vi "Preprocess_and_Convert_IMAQ_Image_to_Array.vi"(7 "PreProcessing_Options":T2={"DS_Name"="delete", "Input_Dims"={"C"=3, "H"=224, "W"=224}, "Center Crop Size"=0, "Interpolation Type"=1, "Multi-Stage_DownSample?"=FALSE, "Dataset_Stats"={"means"={"R"=0.5385, "G"=0.5348, "B"=0.551}, "stds"={"R"=0.3673, "G"=0.3673, "B"=0.3505}}} {"Dataset_Stats"."stds"."R" format="%#_3g"; "Dataset_Stats"."stds"."G" format="%#_3g"; "Dataset_Stats"."stds"."B" format="%#_3g"; "Dataset_Stats"."means"."R" format="%#_3g"; "Dataset_Stats"."means"."G" format="%#_3g"; "Dataset_Stats"."means"."B" format="%#_3g"; "Interpolation Type" items=["Zero Order", "Bi-Linear", "Quadratic", "Cubic Spline"]}, 8 "error in (no error)":errorcluster, 11 "Imaq Image In":T1=refnum) -> (0 "error out":errorcluster, 2 "Norm_Img_Out":sgl[][][](array[numeric]), 3 "Imaq Image Out":T1, 5 "dT_Preprocessing":dbl=0.0017125000013038516)   [LabVIEW 2024]
uses:
  <vilib>/Ngene/DeepLTK Anomaly Detection Addon/DeepLTK_Anomaly_Detection_Addon/API/Controls/NNPC_PreProcessing_Options.ctl
  <vilib>/Ngene/Deep Learning Toolkit/Toolkit/NN_Data/API/NN_Dims(C,H,W).ctl
  <vilib>/Ngene/DeepLTK Anomaly Detection Addon/DeepLTK_Anomaly_Detection_Addon/API/Controls/NNPC_DS_Stats.ctl
  <vilib>/Ngene/DeepLTK Anomaly Detection Addon/DeepLTK_Anomaly_Detection_Addon/API/Controls/Image_Stats_RGB.ctl
  <vilib>/vision/Image Controls.llb/IMAQ Image.ctl
  <vilib>/vision/NI_Vision_Development_Module.lvlib
  <vilib>/Ngene/Deep Learning Toolkit/Toolkit/Deep_Learning_Toolkit_by_Ngene.lvlib
  <vilib>/Ngene/DeepLTK Anomaly Detection Addon/DeepLTK_Anomaly_Detection_Addon/DeepLTK_Anomaly_Detection_Addon.lvlib
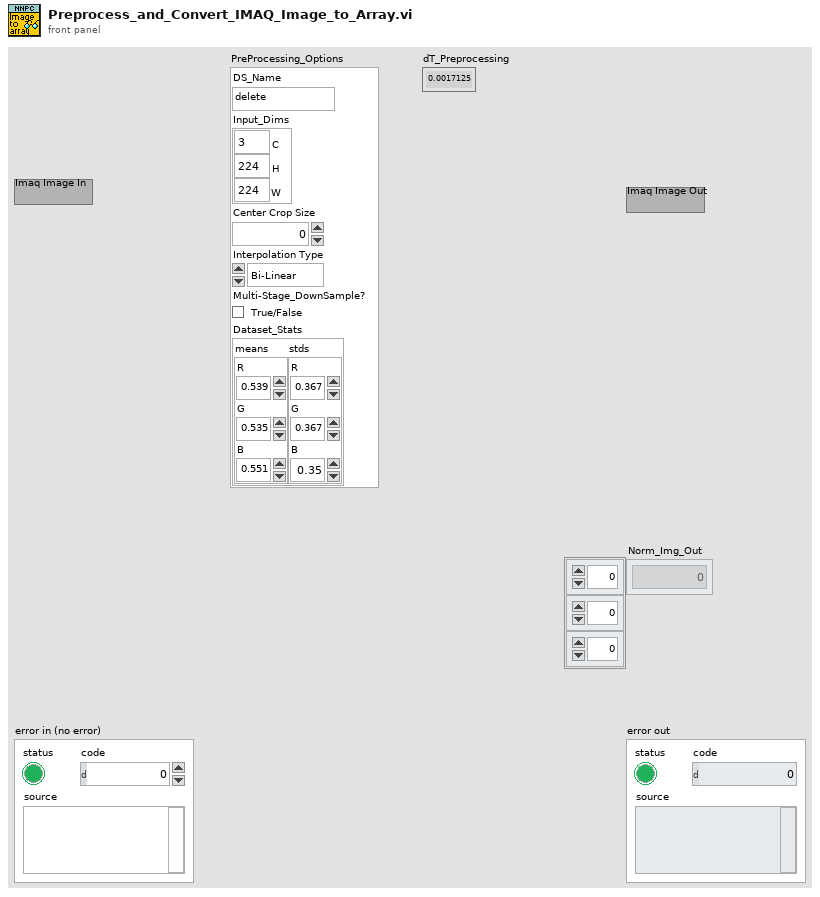
[diagram p1: front panel]
types:
  T1 = typedef "IMAQ Image.ctl" = refnum<image>
  T2 = typedef "DeepLTK_Anomaly_Detection_Addon.lvlib/NNPC_PreProcessing_Options.ctl" = cluster{"DS_Name":string, "Input_Dims":T3, "Center Crop Size":i32, "Interpolation Type":u32, "Multi-Stage_DownSample?":bool, "Dataset_Stats":T4}
  T3 = typedef "Deep_Learning_Toolkit_by_Ngene.lvlib/NN_Dims(C,H,W).ctl" = cluster{"C":i32, "H":i32, "W":i32}
  T4 = typedef "DeepLTK_Anomaly_Detection_Addon.lvlib/NNPC_DS_Stats.ctl" = cluster{"means":T5, "stds":T5}
  T5 = typedef "DeepLTK_Anomaly_Detection_Addon.lvlib/Image_Stats_RGB.ctl" = cluster{"R":sgl, "G":sgl, "B":sgl}
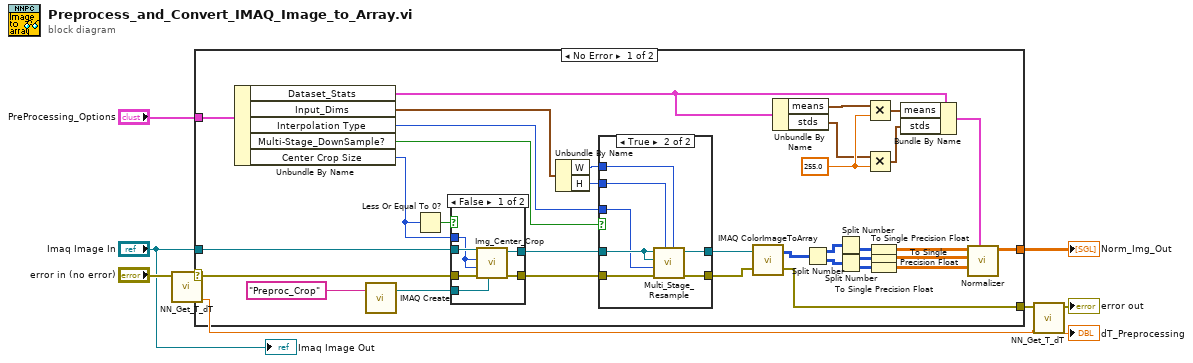
[diagram p0: block diagram]
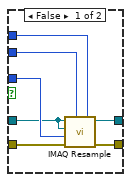
[diagram p2: hidden frame]
diagram:
  n1 = call <vilib>:"NN_Get_T_dT.vi"("error in (no error)"="error in (no error)") -> ("T_out"=w2:dbl, "error out"=w3:errorcluster)  [unwired: 6 in, 1 out]
  n2 = case shown="No Error" w3 {
    selector: w3 -> [w19 w66]
    tunnel: "PreProcessing_Options" -> [w43 _]
    tunnel: "Imaq Image In" -> [w18 _]
    tunnel: [w21 w66] -> w8
    tunnel: [w20 _] -> w7
    frame No Error {
      w35 = sgl 255.0 ("R")
      n3 = Unbundle By Name(w43) -> ("Dataset_Stats"=w36:T4, "Input_Dims"=w26:T3, "Interpolation Type"=w13:u32, "Multi-Stage_DownSample?"=w12:bool, "Center Crop Size"=w14:i32)
      n4 = call "IMAQ Create"("Image Name"="Preproc_Crop") -> ("New Image"=w10:T1)  [unwired: 4 in, 1 out]
      n5 = Less Or Equal To 0?(x=w14) -> (x <= 0?=w15:bool)
      n6 = case shown="False" w15 {
        tunnel: w18 -> [w63 w65]
        tunnel: [w62 w65] -> w17
        tunnel: w19 -> [w61 w64]
        tunnel: [w60 w64] -> w16
        tunnel: w14 -> [w59 _]
        tunnel: w10 -> [w58 _]
        frame False {
          n7 = call "Img_Center_Crop.vi"("Image Dst"=w58, "error in (no error)"=w61, "height"=w59, "width"=w59, "Image In"=w63) -> ("error out"=w60:errorcluster, "Image Out"=w62:T1)  [unwired: 5 in]
        }
        frame True {
        }
      }
      n8 = Unbundle By Name(w26) -> ("W"=w24:i32, "H"=w23:i32)
      n9 = case shown="True" w12 {
        tunnel: [w50 w54] -> w25
        tunnel: [w49 w55] -> w22
        tunnel: w13 -> [w48 w51]
        tunnel: w17 -> [w44 w52]
        tunnel: w24 -> [w47 w53]
        tunnel: w23 -> [w46 w56]
        tunnel: w16 -> [w45 w57]
        frame False {
          n10 = call "IMAQ Resample"("X Resolution"=w47, "Y Resolution"=w46, "error in (no error)"=w45, "Interpolation Type"=w48, "Image Dst"=w44, "Image Src"=w44) -> ("error out"=w50:errorcluster, "Image Dst Out"=w49:T1)  [unwired: 4 in]
        }
        frame True {
          n11 = call "Multi_Stage_Resample.vi"("X Resolution"=w53, "Y Resolution"=w56, "error in (no error)"=w57, "Interpolation Type"=w51, "Img in"=w52, "Dest"=w52) -> ("error out"=w54:errorcluster, "Img out"=w55:T1)  [unwired: 4 in]
        }
      }
      n12 = call "IMAQ ColorImageToArray"("Image"=w22, "error in (no error)"=w25) -> ("Image Pixels (U32)"=w32:u32[][], "error out"=w21:errorcluster)  [unwired: 2 in, 1 out]
      n13 = Unbundle By Name(w36) -> ("means"=w33:T5, "stds"=w34:T5)
      n14 = Split Number(x=w32) -> (hi(x)=w28:u16[][], lo(x)=w27:u16[][])
      n15 = Split Number(x=w28) -> (lo(x)=w29:u8[][])  [unwired: 1 out]
      n16 = Split Number(x=w27) -> (hi(x)=w30:u8[][], lo(x)=w31:u8[][])
      n17 = Multiply(x=w33, y=w35) -> (x*y=w38:T5)
      n18 = Multiply(x=w34, y=w35) -> (x*y=w39:T5)
      n19 = To Single Precision Float(number=w29) -> (single precision float=w40:sgl[][])
      n20 = To Single Precision Float(number=w30) -> (single precision float=w41:sgl[][])
      n21 = To Single Precision Float(number=w31) -> (single precision float=w42:sgl[][])
      n22 = Bundle By Name(cluster=w36, "means"=w38, "stds"=w39) -> (w37:T4)
      n23 = call "Normalizer.vi"("Dataset_Stats"=w37, "B"=w42, "G"=w41, "R"=w40) -> ("Norm_Img_Out"=w20:sgl[][][])  [unwired: 7 in]
    }
    frame Error {
    }
  }
  "Norm_Img_Out" <- w7
  n24 = call <vilib>:"NN_Get_T_dT.vi"("T_in"=w2, "error in (no error)"=w8) -> ("error out"=→"error out":errorcluster, "dT"=→"dT_Preprocessing":dbl)  [unwired: 5 in, 1 out]
  "Imaq Image Out" <- "Imaq Image In"
